vi "DemoGUI.vi"() -> ()   [LabVIEW 2013]
uses:
  C:/Program Files (x86)/LabNation/SmartScope/DeviceInterface.dll
  Program Files (x86)/LabNation/SmartScope/DeviceInterface.dll
panel:
  in  "ChB Offset":dbl(slide)=2.0 scale=-4.0..4.0
  in  "ChB V/div":i8(knob)=5 caption="Knob" scale=0.0..7.0
  in  "TriggerHoldoff":dbl(slide) scale=-5e-05..5e-05
  in  "Time/div":i8(knob)=6 caption="Knob" scale=0.0..12.0
  in  "ChA Offset":dbl(slide) scale=-4.0..4.0
  in  "ChA V/div":i8(knob)=5 caption="Knob" scale=0.0..7.0
  in  "TriggerLevel":dbl(slide) scale=-4.0..4.0 scale format="%#_6f"
  out "Waveform Graph":dbl[][](graph)
  out "Connected":bool
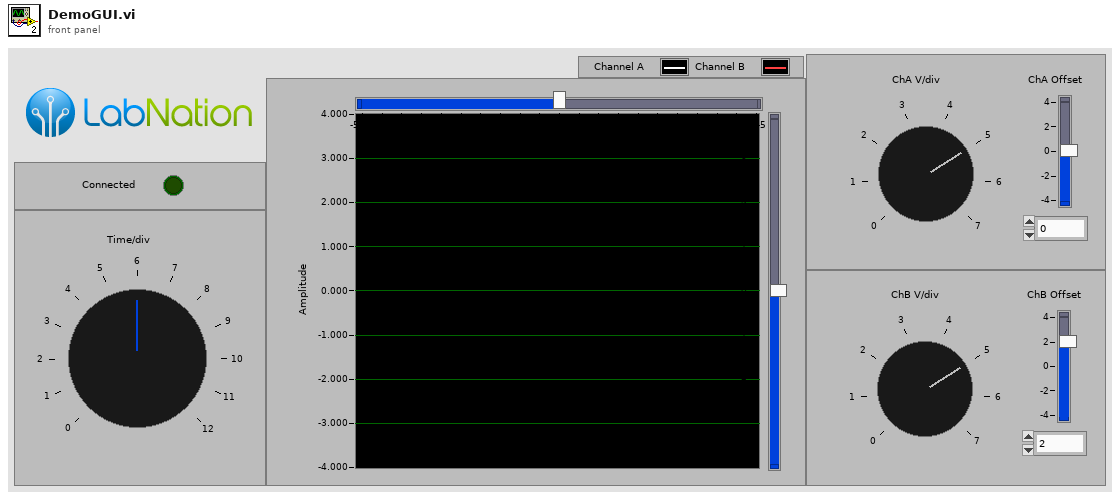
[diagram p1: front panel]
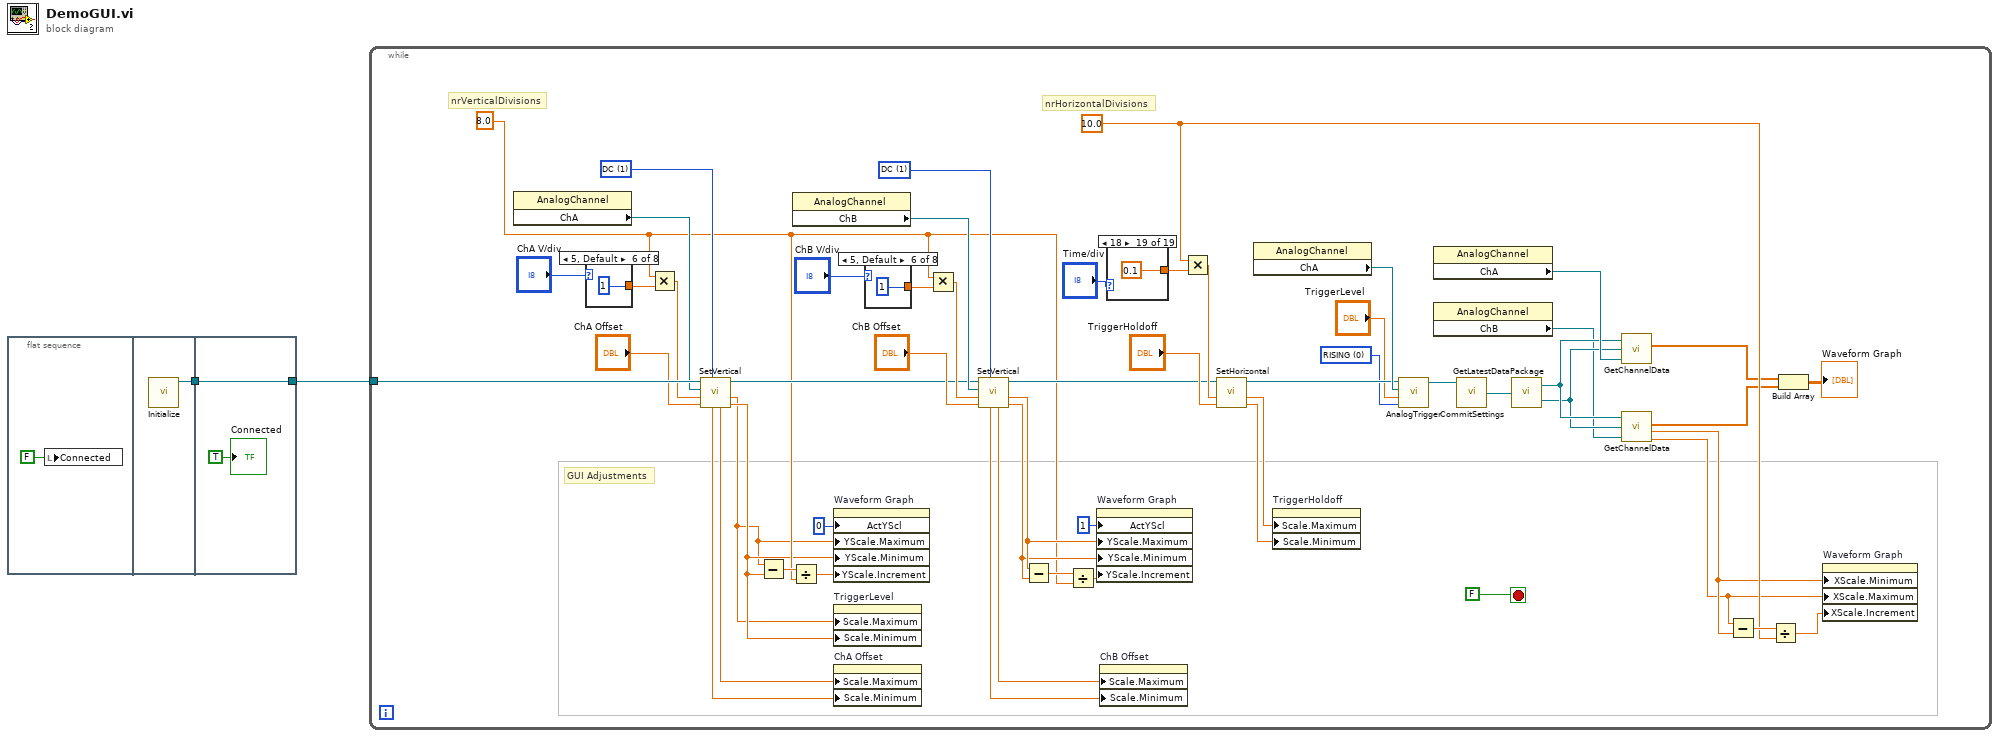
[diagram p0: block diagram]
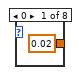
[diagram p2: hidden frame]
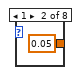
[diagram p3: hidden frame]
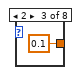
[diagram p4: hidden frame]
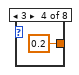
[diagram p5: hidden frame]
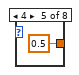
[diagram p6: hidden frame]
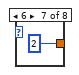
[diagram p7: hidden frame]
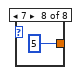
[diagram p8: hidden frame]
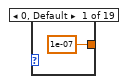
[diagram p9: hidden frame]
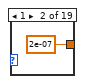
[diagram p10: hidden frame]
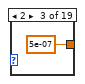
[diagram p11: hidden frame]
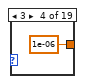
[diagram p12: hidden frame]
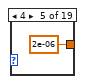
[diagram p13: hidden frame]
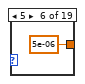
[diagram p14: hidden frame]
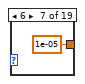
[diagram p15: hidden frame]
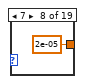
[diagram p16: hidden frame]
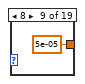
[diagram p17: hidden frame]
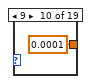
[diagram p18: hidden frame]
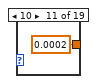
[diagram p19: hidden frame]
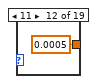
[diagram p20: hidden frame]
diagram:
  n1 = flat-sequence {
    tunnel: [w4] -> w1
    tunnel: [w6] -> w2
    tunnel: w1 -> [w6]
    frame #0 {
      n2 = local write "Connected"(FALSE ("Connected")) -> ()
    }
    frame #1 {
      n3 = call "Initialize.vi"() -> ("LabNation.DeviceInterface.Devices.IScope"=w4:refnum<k24>)  [unwired: 1 in]
    }
    frame #2 {
      "Connected" <- TRUE ("Connected")
    }
  }
  n4 = while {
    tunnel: w2 -> [w58]
    stop <- FALSE stop-if-true
    w34 = 1 items=["AC", "DC"] ("coupling")
    w8 = 0 items=["RISING", "FALLING", "ANY"] ("edge")
    w45 = 1 items=["AC", "DC"] ("coupling")
    w39 = 10.0 ("y")
    w25 = 8.0 ("y")
    # "GUI Adjustments"
    # "nrHorizontalDivisions"
    # "nrVerticalDivisions"
    n5 = property class="AnalogChannel"() -> ("ChA"=w53:refnum<k24>)  [unwired: 2 in, 2 out]
    n6 = case shown="5, Default" "ChA V/div" {
      tunnel: [0.02 0.05 0.1 0.2 0.5 1 2 5] -> w44
      frame 0 {
      }
      frame 1 {
      }
      frame 2 {
      }
      frame 3 {
      }
      frame 4 {
      }
      frame 5, Default {
      }
      frame 6 {
      }
      frame 7 {
      }
    }
    n7 = Multiply(x=w25, y=w44) -> (x*y=w55:dbl)
    n8 = call "SetVertical.vi"("coupling"=w45, "Offset"="ChA Offset", "Range"=w55, "LabNation.DeviceInterface.Devices.AnalogChannel"=w53, "LabNation.DeviceInterface.Devices.IScope"=w58) -> ("GraphMin"=w22:dbl, "GraphMax"=w21:dbl, "LabNation.DeviceInterface.Devices.IScope"=w32:refnum<k24>, "OffsetMax"=w57:dbl, "OffsetMin"=w56:dbl)  [unwired: 2 in]
    n9 = Subtract(x=w21, y=w22) -> (x-y=w46:dbl)
    n10 = Divide(x=w46, y=w25) -> (x/y=w23:dbl)
    n11 = property class="AnalogChannel"() -> ("ChB"=w35:refnum<k24>)  [unwired: 2 in, 2 out]
    n12 = property on="Waveform Graph" class="WFGraph (strict)"("ActYScl"=0 ("Active Y Scale"), "YScale.Maximum"=w21, "YScale.Minimum"=w22, "YScale.Increment"=w23) -> ()  [unwired: 2 in, 2 out]
    n13 = property on="TriggerLevel" class="Slide (strict)"("Scale.Maximum"=w21, "Scale.Minimum"=w22) -> ()  [unwired: 2 in, 2 out]
    n14 = property on="ChA Offset" class="Slide (strict)"("Scale.Maximum"=w57, "Scale.Minimum"=w56) -> ()  [unwired: 2 in, 2 out]
    n15 = case shown="5, Default" "ChB V/div" {
      tunnel: [0.02 0.05 0.1 0.2 0.5 1 2 5] -> w33
      frame 0 {
      }
      frame 1 {
      }
      frame 2 {
      }
      frame 3 {
      }
      frame 4 {
      }
      frame 5, Default {
      }
      frame 6 {
      }
      frame 7 {
      }
    }
    n16 = Multiply(x=w25, y=w33) -> (x*y=w37:dbl)
    n17 = call "SetVertical.vi"("coupling"=w34, "Offset"="ChB Offset", "Range"=w37, "LabNation.DeviceInterface.Devices.AnalogChannel"=w35, "LabNation.DeviceInterface.Devices.IScope"=w32) -> ("GraphMin"=w27:dbl, "GraphMax"=w28:dbl, "LabNation.DeviceInterface.Devices.IScope"=w31:refnum<k24>, "OffsetMax"=w19:dbl, "OffsetMin"=w18:dbl)  [unwired: 2 in]
    n18 = Subtract(x=w28, y=w27) -> (x-y=w26:dbl)
    n19 = Divide(x=w26, y=w25) -> (x/y=w24:dbl)
    n20 = property on="Waveform Graph" class="WFGraph (strict)"("ActYScl"=u32 1 ("Plot.Y Scale Index"), "YScale.Maximum"=w28, "YScale.Minimum"=w27, "YScale.Increment"=w24) -> ()  [unwired: 2 in, 2 out]
    n21 = property on="ChB Offset" class="Slide (strict)"("Scale.Maximum"=w19, "Scale.Minimum"=w18) -> ()  [unwired: 2 in, 2 out]
    n22 = case shown="18" "Time/div" {
      tunnel: [1e-07 2e-07 5e-07 1e-06 2e-06 5e-06 1e-05 2e-05 5e-05 0.0001 0.0002 0.0005 0.001 0.002 0.005 0.01 0.02 0.05 0.1] -> w43
      frame 0, Default {
      }
      frame 1 {
      }
      frame 2 {
      }
      frame 3 {
      }
      frame 4 {
      }
      frame 5 {
      }
      frame 6 {
      }
      frame 7 {
      }
      frame 8 {
      }
      frame 9 {
      }
      frame 10 {
      }
      frame 11 {
      }
      frame 12 {
      }
      frame 13 {
      }
      frame 14 {
      }
      frame 15 {
      }
      frame 16 {
      }
      frame 17 {
      }
      frame 18 {
      }
    }
    n23 = Multiply(x=w39, y=w43) -> (x*y=w49:dbl)
    n24 = call "SetHorizontal.vi"("TriggerHoldoff"="TriggerHoldoff", "ViewportLength"=w49, "LabNation.DeviceInterface.Devices.IScope"=w31) -> ("TrigSliderMin"=w50:dbl, "TrigSliderMax"=w51:dbl, "LabNation.DeviceInterface.Devices.IScope"=w41:refnum<k24>)  [unwired: 2 in]
    n25 = property class="AnalogChannel"() -> ("ChA"=w42:refnum<k24>)  [unwired: 2 in, 2 out]
    n26 = property on="TriggerHoldoff" class="Slide (strict)"("Scale.Maximum"=w51, "Scale.Minimum"=w50) -> ()  [unwired: 2 in, 2 out]
    n27 = call "AnalogTrigger.vi"("EdgeType"=w8, "TriggerLevel"="TriggerLevel", "LabNation.DeviceInterface.Devices.AnalogChannel"=w42, "LabNation.DeviceInterface.Devices.IScope"=w41) -> ("LabNation.DeviceInterface.Devices.IScope"=w40:refnum<k24>)
    n28 = property class="AnalogChannel"() -> ("ChA"=w16:refnum<k24>)  [unwired: 2 in, 2 out]
    n29 = property class="AnalogChannel"() -> ("ChB"=w13:refnum<k24>)  [unwired: 2 in, 2 out]
    n30 = call "CommitSettings.vi"("LabNation.DeviceInterface.Devices.IScope"=w40) -> ("LabNation.DeviceInterface.Devices.IScope"=w17:refnum<k24>)
    n31 = call "GetLatestDataPackage.vi"("LabNation.DeviceInterface.Devices.IScope"=w17) -> ("LabNation.DeviceInterface.Devices.IScope"=w15:refnum<k24>, "LabNation.DeviceInterface.DataSources.DataPackageScope"=w14:refnum<k24>)
    n32 = call "GetChannelData.vi"("LabNation.DeviceInterface.Devices.IScope"=w15, "LabNation.DeviceInterface.DataSources.DataPackageScope"=w14, "AnalogChannel"=w16) -> ("Waveform Graph"=w12:dbl[])  [unwired: 3 out]
    n33 = call "GetChannelData.vi"("LabNation.DeviceInterface.Devices.IScope"=w15, "LabNation.DeviceInterface.DataSources.DataPackageScope"=w14, "AnalogChannel"=w13) -> ("Waveform Graph"=w11:dbl[], "ViewportBegin"=w10:dbl, "ViewportEnd"=w9:dbl)  [unwired: 1 out]
    n34 = Subtract(x=w9, y=w10) -> (x-y=w48:dbl)
    n35 = Divide(x=w48, y=w39) -> (x/y=w47:dbl)
    n36 = Build Array(w12, w11) -> (→"Waveform Graph":dbl[][])
    n37 = property on="Waveform Graph" class="WFGraph (strict)"("XScale.Minimum"=w10, "XScale.Maximum"=w9, "XScale.Increment"=w47) -> ()  [unwired: 2 in, 2 out]
  }
